vi "Shooter Control PID.vi"(4 "Low Stop-Band":dbl=6.0, 5 "High Stop-Band":dbl=1.5, 6 "PID gains":T1={"proportional gain (Kc)"=0.165, "integral time (Ti, min)"=0.0, "derivative time (Td, min)"=0.0}, 7 "PID Vision gains":T1={"proportional gain (Kc)"=1.3, "integral time (Ti, min)"=0.0, "derivative time (Td, min)"=0.0}, 9 "Angle Based Deadband":dbl=7.0, 10 "In Deadband Strength":dbl=0.5, 11 "y":dbl=0.08) -> (2 "Manual Limit Override":bool, 3 "Shooter Rotation Angle":dbl=57.60243247876565)   [LabVIEW 2012]
uses:
  <vilib>/Rock Robotics/WPI/DriverStation/DriverStationLCD/WPI_DriverStationLCDLCDLine.ctl
  Users/developer/Desktop/Post TCNJ/Robot Global Data.vi
  <vilib>/addons/control/pid/pid.llb/PID (DBL).vi
  <vilib>/addons/control/pid/NI_PID_pid.lvlib
panel:
  in  "x":dbl=0.2
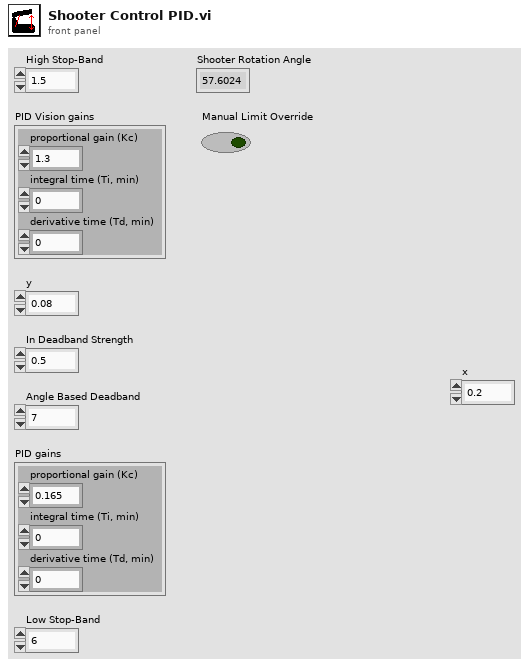
[diagram p1: front panel]
types:
  T1 = cluster{"proportional gain (Kc)":dbl, "integral time (Ti, min)":dbl, "derivative time (Td, min)":dbl}
  T2 = typedef "WPI_DriverStationLCDLCDLine.ctl" = enum16{"Main - Line 1", "User - Line 2", "User - Line 3", "User - Line 4", "User - Line 5", "User - Line 6"}
  T3 = typedef "WPI_MotorControlDeviceRef.ctl" = cluster{"DeviceStatus":errorcluster, "Type":enum16{"PWM", "CAN"}, "PWM":cluster{"Digital Module":T4, "PWM Channel":T5, "DeadBand":T6}, "CAN":cluster{"Device Number":u8, "Control Mode":T7, "Semaphore":T8, "Max Vout":dbl}, "Invert":bool, "TransformRef":T9, "InvTransformRef":T9}
  T4 = typedef "FPGA_TypedefDigitalModule.ctl" = enum16{"Digital Module 1", "Digital Module 2"}
  T5 = typedef "FPGA_DIOPWMChannel.ctl" = enum8{"PWM 1", "PWM 2", "PWM 3", "PWM 4", "PWM 5", "PWM 6", "PWM 7", "PWM 8", "PWM 9", "PWM 10", "Invalid"}
  T6 = typedef "WPI_PWMDeadband.ctl" = cluster{"Name":string, "maxPositivePwm":i32, "minPositivePwm":i32, "centerPwm":i32, "maxNegativePwm":i32, "minNegativePwm":i32, "angularRange":u16}
  T7 = typedef "WPI_CANJaguar_ControlMode.ctl" = enum8{"Percent VBus", "Current", "Speed", "Position", "Voltage"}
  T8 = typedef "Semaphore RefNum" = refnum<k1>
  T9 = typedef "WPI_PWMTransform_ConPane.ctl" = refnum<vi>
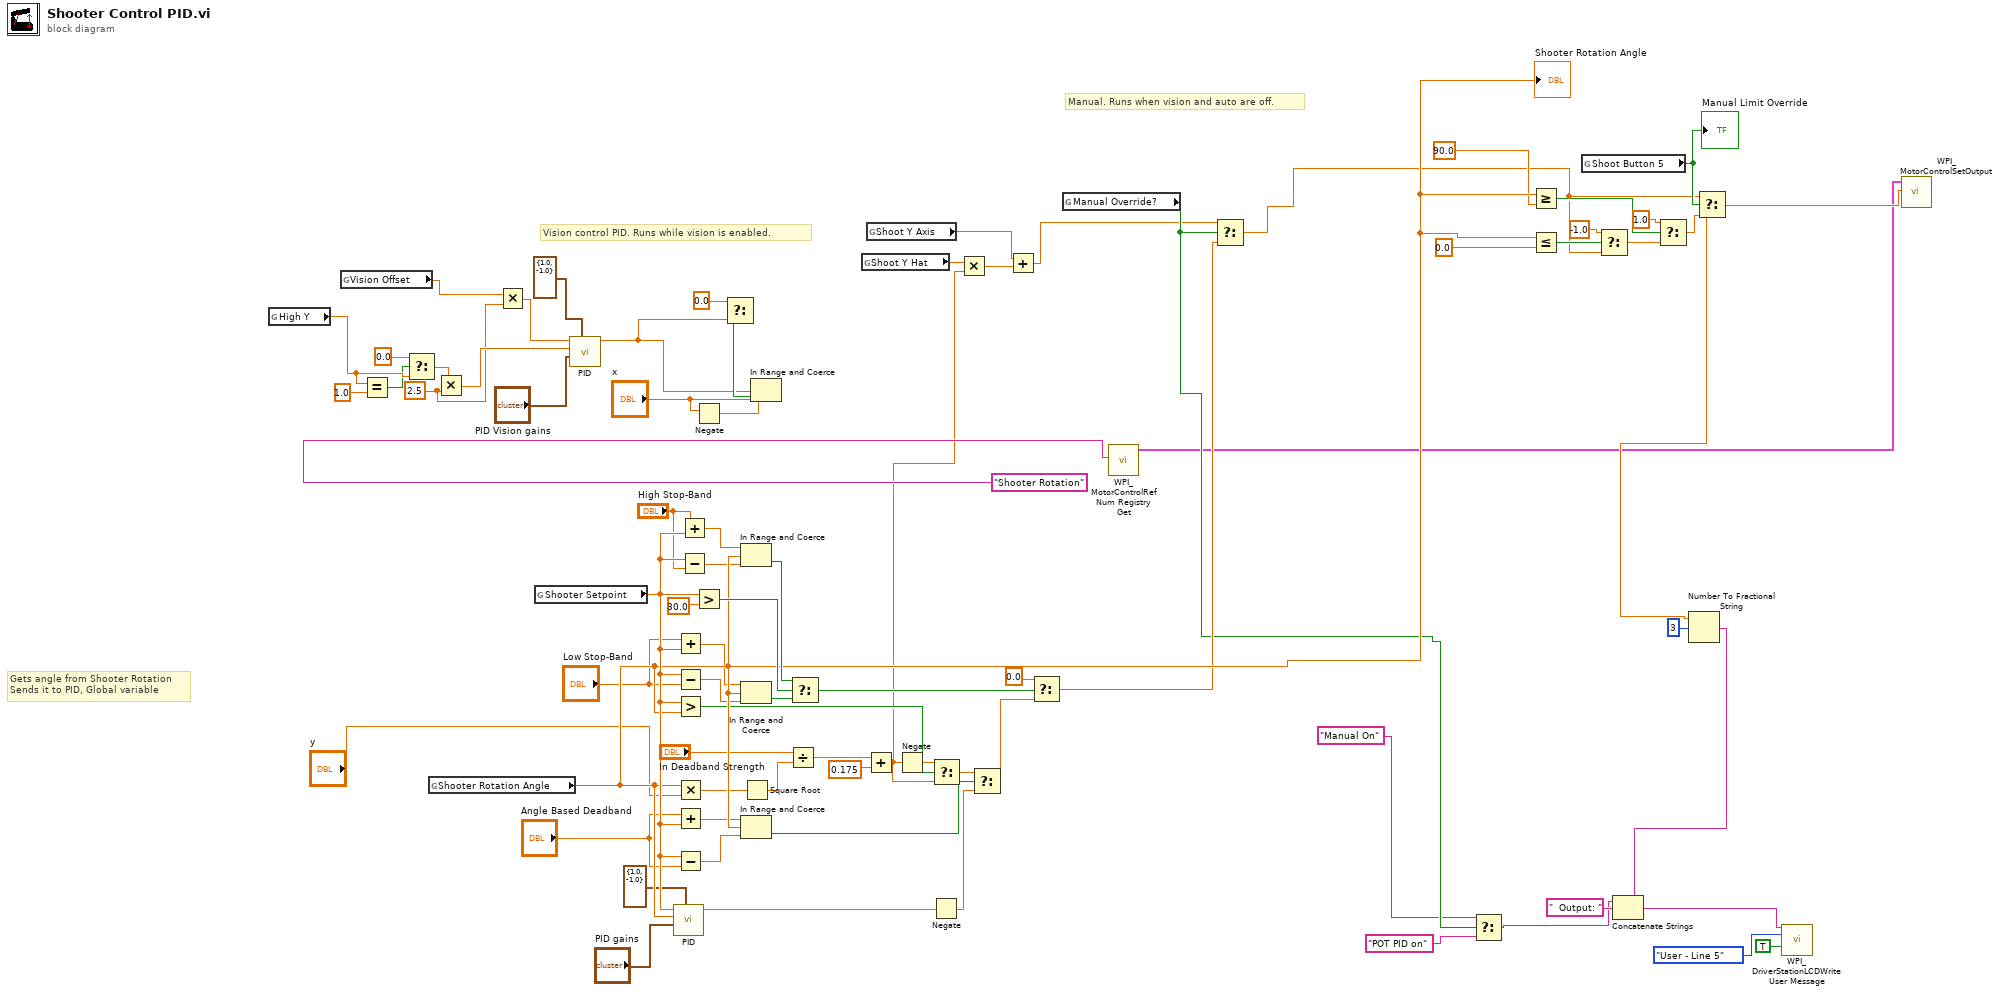
[diagram p0: block diagram]
diagram:
  w41 = 2.5 ("y")
  # "Manual. Runs when vision and auto are off."
  # "Vision control PID. Runs while vision is enabled."
  # "Gets angle from Shooter Rotation\nSends it to PID, Global variable"
  n1 = global read "Robot Global Data.vi" "High Y"() -> (w46:dbl)
  n2 = global read "Robot Global Data.vi" "Vision Offset"() -> (w44:dbl)
  n3 = Equal?(x=w46, y=1.0) -> (x = y?=w45:bool)
  n4 = Select(t=0.0, s=w45, f=w46) -> (s? t:f=w40:dbl)
  n5 = global read "Robot Global Data.vi" "Shooter Rotation Angle"() -> (w68:dbl)
  "Shooter Rotation Angle" <- w68
  n6 = Multiply(x=w40, y=w41) -> (x*y=w43:dbl)
  n7 = Multiply(x=w44, y=w41) -> (x*y=w42:dbl)
  n8 = global read "Robot Global Data.vi" "Shooter Setpoint"() -> (w73:dbl)
  n9 = call-poly <vilib>:"PID.vi"("output range"=cluster{"output high":dbl, "output low":dbl} {"output high"=1.0, "output low"=-1.0}, "PID gains"="PID Vision gains", "process variable"=w43, "setpoint"=w42) -> ("output"=w6:dbl)  [unwired: 6 in, 1 out]
  n10 = call-poly <vilib>:"PID.vi"("output range"=cluster{"output high":dbl, "output low":dbl} {"output high"=1.0, "output low"=-1.0}, "PID gains"="PID gains", "process variable"=w68, "setpoint"=w73) -> ("output"=w19:dbl)  [unwired: 6 in, 1 out]
  n11 = Add(x="Low Stop-Band", y=w73) -> (x+y=w65:dbl)
  n12 = Subtract(x=w73, y="Low Stop-Band") -> (x-y=w66:dbl)
  n13 = Greater?(x=w73, y=w68) -> (0:w52:bool)
  n14 = Multiply(x=w68, y="y") -> (x*y=w63:dbl)
  n15 = Add(x="Angle Based Deadband", y=w73) -> (x+y=w47:dbl)
  n16 = Subtract(x=w73, y="Angle Based Deadband") -> (x-y=w49:dbl)
  n17 = Add(x="High Stop-Band", y=w73) -> (x+y=w55:dbl)
  n18 = Subtract(x=w73, y="High Stop-Band") -> (x-y=w56:dbl)
  n19 = Negate(x="x") -> (-x=w3:dbl)
  n20 = Greater?(x=w73, y=30.0) -> (0:w72:bool)
  n21 = In Range and Coerce(upper limit=w55, x=w68, lower limit=w56) -> (In Range?=w69:bool)  [unwired: 1 out]
  n22 = In Range and Coerce(upper limit=w65, x=w68, lower limit=w66) -> (In Range?=w70:bool)  [unwired: 1 out]
  n23 = In Range and Coerce(upper limit=w47, x=w68, lower limit=w49) -> (In Range?=w50:bool)  [unwired: 1 out]
  n24 = Square Root(x=w63) -> (sqrt(x)=w64:dbl)
  n25 = In Range and Coerce(upper limit="x", x=w6, lower limit=w3) -> (In Range?=w7:bool)  [unwired: 1 out]
  n26 = Select(t=0.0, s=w7, f=w6) -> ()  [unwired: 1 out]
  n27 = Divide(x="In Deadband Strength", y=w64) -> (x/y=w14:dbl)
  n28 = Select(t=w69, s=w72, f=w70) -> (s? t:f=w71:bool)
  n29 = global read "Robot Global Data.vi" "Shoot Y Hat"() -> (w12:dbl)
  n30 = global read "Robot Global Data.vi" "Shoot Y Axis"() -> (w10:dbl)
  n31 = Add(x=w14, y=0.175) -> (x+y=w11:dbl)
  n32 = Negate(x=w11) -> (-x=w54:dbl)
  n33 = Negate(x=w19) -> (-x=w51:dbl)
  n34 = Select(t=w54, s=w52, f=w11) -> (s? t:f=w53:dbl)
  n35 = Multiply(x=w12, y=w11) -> (x*y=w9:dbl)
  n36 = Select(t=w53, s=w50, f=w51) -> (s? t:f=w58:dbl)
  n37 = Add(x=w10, y=w9) -> (x+y=w8:dbl)
  n38 = Select(t=0.0, s=w71, f=w58) -> (s? t:f=w60:dbl)
  n39 = global read "Robot Global Data.vi" "Manual Override?"() -> (w33:bool)
  n40 = call <vilib>:"WPI_MotorControlRefNum Registry Get.vi"("refnum name"="Shooter Rotation") -> ("MotorControlDevRef"=w16:T3)  [unwired: 9 in, 1 out]
  n41 = Select(t=w8, s=w33, f=w60) -> (s? t:f=w2:dbl)
  n42 = Select(t="Manual On", s=w33, f="POT PID on") -> (s? t:f=w1:string)
  n43 = Greater Or Equal?(x=w68, y=90.0 ("upper limit")) -> (x >= y?=w23:bool)
  n44 = Less Or Equal?(x=w68, y=0.0 ("lower limit")) -> (x <= y?=w24:bool)
  n45 = global read "Robot Global Data.vi" "Shoot Button 5"() -> (w30:bool)
  "Manual Limit Override" <- w30
  n46 = Select(t=-1.0, s=w24, f=w2) -> (s? t:f=w28:dbl)
  n47 = Select(t=1.0, s=w23, f=w28) -> (s? t:f=w29:dbl)
  n48 = Select(t=w2, s=w30, f=w29) -> (s? t:f=w75:dbl)
  n49 = Number To Fractional String(number=w75, width (-)=i16 3) -> (F-format string=w76:string)  [unwired: 2 in]
  n50 = Concatenate Strings(w1, "  Output: " ("string"), w76) -> (w37:string)
  n51 = call <vilib>:"WPI_DriverStationLCDWrite User Message.vi"("line text"=w37, "line"=WPI_DriverStationLCDLCDLine."User - Line 5", "clear line before write (T)"=TRUE) -> ()  [unwired: 12 in, 1 out]
  n52 = call <vilib>:"WPI_MotorControlSetOutput.vi"("Output"=w75, "MotorControlDevRef"=w16) -> ()  [unwired: 7 in, 3 out]
